vi "Elevator Idle Trashcan Stabilizer.vi"(9 "Tote Count":i32, 10 "Has Trashcan?":bool, 11 "Elevator in position?":bool) -> (3 "Close stabilizer":bool)   [LabVIEW 2014]
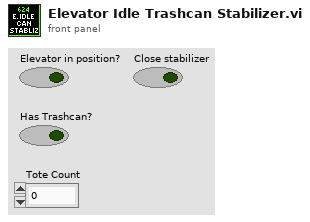
[diagram p1: front panel]
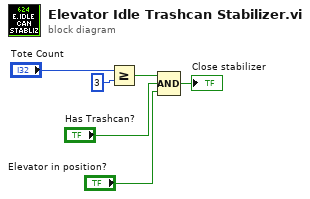
[diagram p0: block diagram]
diagram:
  n1 = Greater Or Equal?(x="Tote Count", y=3) -> (x >= y?=w2:bool)
  n2 = Compound Arithmetic op=AND(w2, "Has Trashcan?", "Elevator in position?") -> (→"Close stabilizer":bool)
